vi "clearpath_set_velocity.vi"(0 "ClearpathComm":T1, 1 "Zero Speeds":bool=TRUE, 2 "Rotational Speed":dbl, 3 "Translational Speed":dbl) -> ()   [LabVIEW 2012, in "clearpath_interface.lvlib"]
doc: "Formats a Set Velocity command (0x204) given desired translational and rotational speeds (in m/s and rad/s, respectively). The \"Zero Speeds\" flag sets the desired speeds to 0,0. Uses the onboard Clearpath library to perform the actual message formatting."
uses:
  clearpath_interface.lvlib
  cwrap_crio.dll
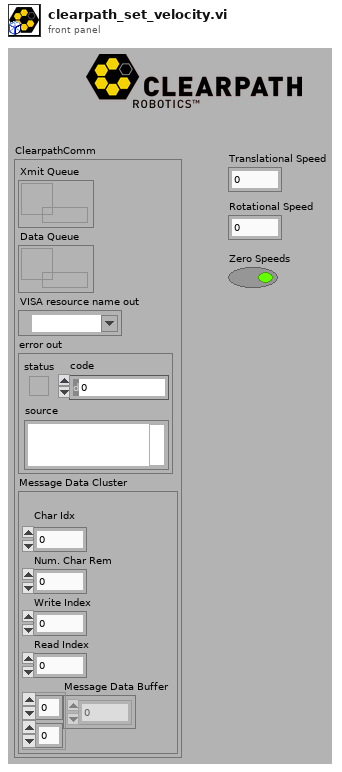
[diagram p1: front panel]
types:
  T1 = cluster{"Xmit Queue":refnum<queue>, "Data Queue":refnum<queue>, "VISA resource name out":refnum<visa-resource-name>, "error out":errorcluster, "Message Data Cluster":cluster{"\nChar Idx":u8, "Num. Char Rem":u8, "Write Index":u8, "Read Index":u8, "Message Data Buffer":u8[][]}}
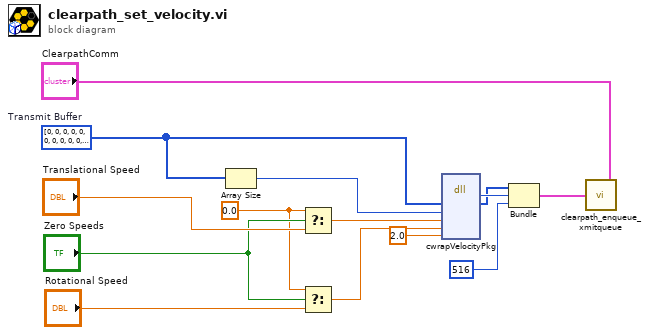
[diagram p0: block diagram]
diagram:
  w8 = 0.0 ("t")
  w10 = u8[] [0, 0, 0, 0, 0, 0, 0, 0, 0, 0, 0, 0, 0, 0, 0, 0, 0, 0, 0, 0, 0, 0, 0, 0, 0, 0, 0, 0, 0, 0, 1, 0, 0, 0, 5]  # Transmit Buffer
  n1 = Array Size(array=w10) -> (size(s)=w9:i32)
  n2 = Select(t=w8, s="Zero Speeds", f="Translational Speed") -> (s? t:f=w6:dbl)
  n3 = Select(t=w8, s="Zero Speeds", f="Rotational Speed") -> (s? t:f=w7:dbl)
  n4 = dll-call lib="C:/Users/cartersm/Documents/GitHub/IGVC-2013/Code/Project 1.0/Motors/Husky/cwrap_cRIO.*" fn="cwrapVelocityPkg"("buf"=w10, "buf_size"=w9, "trans"=w6, "rot"=w7, "accel"=2.0) -> ("return type"=w4:i32, "buf"=w3:u8[])  [unwired: 7 in, 2 out]
  n5 = Bundle("buf"=w3, "return type"=w4, 516) -> (w1:cluster{"buf":u8[], "return type":i32, i32})  [unwired: 1 in]
  n6 = call "clearpath_enqueue_xmitqueue.vi"("ClearpathComm"="ClearpathComm", "Cluster"=w1) -> ()
